vi "global_and_local_image_subtraction_arrays.vi"(9 "Input \nparameters":T4={"Frame rate (ms)"=2000, "Worm strain"="N2", "Time t"=0, "State"=enum."Image acquisition", "Time elapsed"=0.0, "Max_num_runs"=100000, "#TTL"=0, "Time of start TTL"=100000, "Image subtraction value"=0, "Time of last TTL"=0, "Number of Columns"=2, "Number of Rows"=2, "# AdjacentTTL"=0, "Sleep deprivation status"="", "Sleep Detection"=FALSE, "# Sleep detections"=0, "Time of first sleep detection"=0, "Time max # adjacent TTL"=0, "Image t-1"=[], "Image t"=[]} {"Number of Rows" items=["1"=1, "2"=2, "3"=3, "4"=4]; "Number of Columns" items=["1"=1, "2"=2, "3"=3, "4"=4]}, 10 "Deprivation\nparameters":T1={"Frame Row"=0, "Kstd"=40.0, "# Images for\nsleep detection"=10, "Kmean"=1.5, "Start time of sleep detection (images):"=1000, 0, "Length (images)"=3600, "# TTL"=10000, "by x images after first detection"=0, "Between TTL pulses"=0, "\nby x detections"=9, "# Total immobility\n detections"=0.0, "max # adjacent\nTTL"=0.0, "TTL x start\ntime deprivation\n"=0.0, "Max #\nadjacent TTL"=10000, " Ca2+\nmode"=0} {"?" items=["1", "2", "3", "4"]; "Frame Row" items=["1", "2", "3", "4"]}, 11 "State":T5) -> (3 "Image subtraction\narrays":T2)   [LabVIEW 2011]
uses:
  Action-Init-Update-Get.ctl
  state.ctl
panel:
  in  "Image subtraction\narrays":T2
  # "Sleep deprivation settings"
  # "Select deprivation animal"
  # "Row"
  # "Column"
  # "Sleep detection parameters"
  # "Sleep deprivation parameters"
  # "Delay deprivation start:"
  # "Pause deprivation (images):"
  # "Stop deprivation after:"
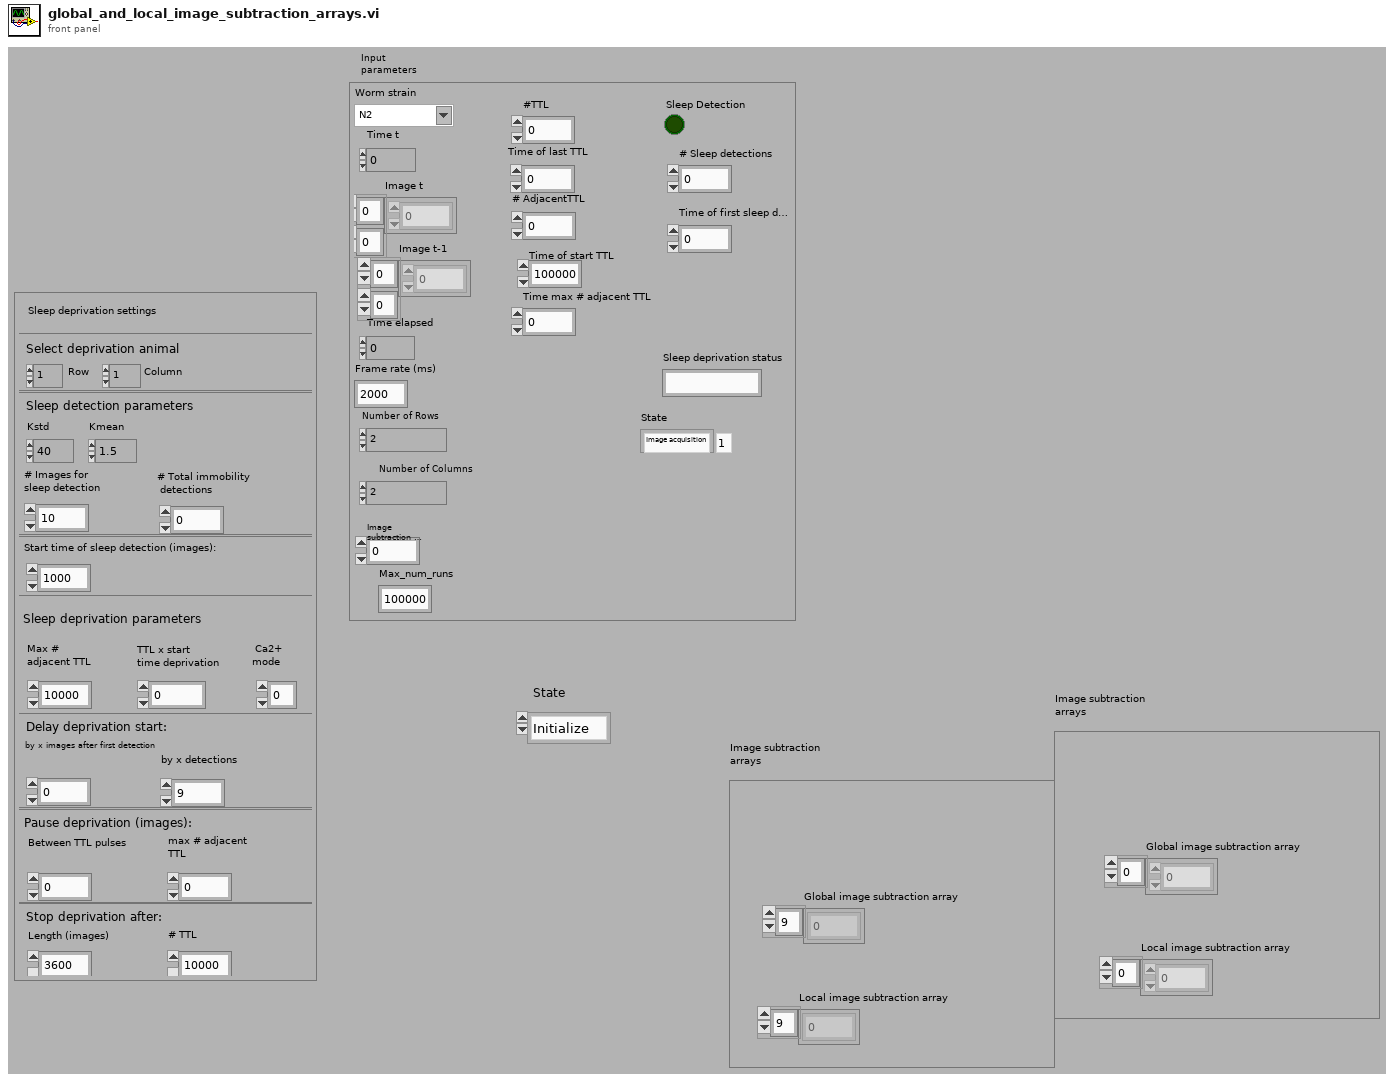
[diagram p1: front panel]
types:
  T1 = cluster{"Frame Row":u32, "Kstd":dbl, "# Images for\nsleep detection":i32, "Kmean":dbl, "Start time of sleep detection (images):":i32, u32, "Length (images)":i32, "# TTL":i32, "by x images after first detection":i32, "Between TTL pulses":i32, "\nby x detections":i32, "# Total immobility\n detections":dbl, "max # adjacent\nTTL":dbl, "TTL x start\ntime deprivation\n":dbl, "Max #\nadjacent TTL":i32, " Ca2+\nmode":i32}
  T2 = cluster{"Global image subtraction array":dbl[], "Local image subtraction array":dbl[]}
  T3 = typedef "state.ctl" = enum16{"Initialize measurement", "Image acquisition", "Image processing", "Sleep detection", "Control TTL protocol ", "Sleep deprivation", "Update image & exit condition", "Wait "}
  T4 = cluster{"Frame rate (ms)":u32, "Worm strain":string, "Time t":i32, "State":T3, "Time elapsed":dbl, "Max_num_runs":i32, "#TTL":i32, "Time of start TTL":i32, "Image subtraction value":i32, "Time of last TTL":i32, "Number of Columns":u32, "Number of Rows":u32, "# AdjacentTTL":i32, "Sleep deprivation status":string, "Sleep Detection":bool, "# Sleep detections":i32, "Time of first sleep detection":i32, "Time max # adjacent TTL":i32, "Image t-1":i32[][], "Image t":i32[][]}
  T5 = typedef "Action-Init-Update-Get.ctl" = enum16{"Initialize", "Update", "Get"}
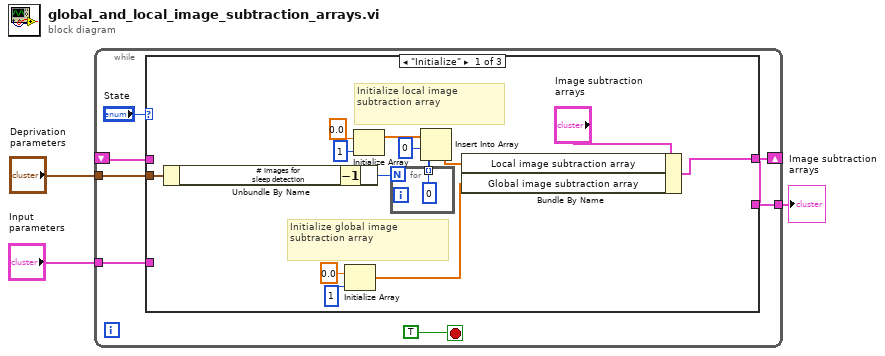
[diagram p0: block diagram]
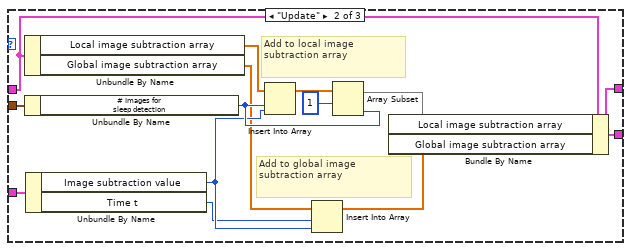
[diagram p2: hidden frame]
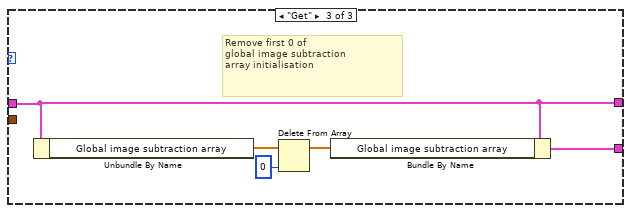
[diagram p3: hidden frame]
diagram:
  n1 = while {
    tunnel: "Input \nparameters" -> [w8]
    shift-right: [w7] -> _
    shift-left: _ -> [w6]
    tunnel: "Deprivation\nparameters" -> [w5]
    tunnel: [w4] -> w1
    stop <- TRUE ("stop") stop-if-true
    n2 = case shown="\"Initialize\"" "State" {
      tunnel: w6 -> [_ w29 w39]
      tunnel: [w11 w26 w39] -> w7
      tunnel: w8 -> [_ w30 _]
      tunnel: w5 -> [w12 w33 _]
      tunnel: [w11 w26 w40] -> w4
      frame "Initialize" {
        # "Initialize global image\nsubtraction array"
        # "Initialize local image\nsubtraction array"
        n3 = Unbundle By Name(w12) -> ("# Images for\nsleep detection"=w16:i32)
        n4 = Decrement(x=w16) -> (x-1=w17:i32)
        n5 = Initialize Array(0.0 ("Element"), 1 ("Index")) -> (w14:dbl[])
        n6 = Initialize Array(0.0 ("Element"), 1 ("Index")) -> (w23:dbl[])
        n7 = for {
          N: w17 -> [_]
          tunnel: [0] -> w18 mode=indexing
        }
        n8 = Insert Into Array(array=w23, index=0 ("Index"), new element=w18) -> (w15:dbl[])
        n9 = Bundle By Name(cluster="Image subtraction\narrays", "Local image subtraction array"=w15, "Global image subtraction array"=w14) -> (w11:T2)
      }
      frame "Update" {
        # "Add to global image \nsubtraction array"
        # "Add to local image \nsubtraction array"
        n10 = Unbundle By Name(w29) -> ("Local image subtraction array"=w28:dbl[], "Global image subtraction array"=w27:dbl[])
        n11 = Unbundle By Name(w33) -> ("# Images for\nsleep detection"=w36:i32)
        n12 = Unbundle By Name(w30) -> ("Image subtraction value"=w35:i32, "Time t"=w34:i32)
        n13 = Insert Into Array(array=w28, index=w36, new element=w35) -> (w38:dbl[])
        n14 = Insert Into Array(array=w27, index=w34, new element=w35) -> (w31:dbl[])
        n15 = Array Subset(array=w38, index=1, length=w36) -> (w32:dbl[])
        n16 = Bundle By Name(cluster=w29, "Local image subtraction array"=w32, "Global image subtraction array"=w31) -> (w26:T2)
      }
      frame "Get" {
        # "Remove first 0 of\nglobal image subtraction\narray initialisation"
        n17 = Unbundle By Name(w39) -> ("Global image subtraction array"=w42:dbl[])
        n18 = Delete From Array(array=w42, index=0) -> (array with subset deleted=w41:dbl[])  [unwired: 1 in, 1 out]
        n19 = Bundle By Name(cluster=w39, "Global image subtraction array"=w41) -> (w40:T2)
      }
    }
  }
  "Image subtraction\narrays" <- w1
